vi "Measurement UI.vi"() -> ()   [LabVIEW 2024, in "Eff And Load Reg_Channel Ganging_UI.lvlib"]
uses:
  Eff And Load Reg_Channel Ganging_UI.lvlib
panel:
  in  "MeasGraphs":T1(tab)
  out "EfficiencyGraph":T2(graph)
  out "LoadRegulationGraph(V/A)":T3(graph)
  out "LoadRegulationGraph(%)":T3(graph)
  out "Load voltage deviation":dbl[](array[numeric])
  out "Ganged load voltages":dbl[](array[numeric])
  in  "Load current pole-zero ratio":dbl=0.3
  in  "Load current compensation frequency":dbl=180000.0
  in  "Load current gain bandwidth":dbl=14000.0
  in  "Source voltage pole-zero ratio":dbl=2.0
  in  "Source voltage compensation frequency":dbl=3530.0
  in  "Source voltage gain bandwidth":dbl=2000.0
  in  "Load slave resource names":string[](array[string])
  in  "Load master resource name":string
  in  "Source slave resource names":string[](array[string])
  in  "Source master resource name":string
  out "Load sweep points":i32
  out "Source sweep points":i32
  out "Voltage values":dbl[](array[numeric])
  out "Efficiency":dbl[](array[numeric])
  out "Ganged load currents":dbl[](array[numeric])
  in  "Mode of operation":T4(ring)=enum."Perform measurement" caption="MODE OF OPERATION"
  in  "MeasConfigurations":T5(tab)=enum."Source Config"
  in  "Nominal output voltage":dbl=1.0 caption="NOMINAL OUTPUT VOLTAGE" format="%.3fV"
  in  "Source delay":dbl=0.005 caption="SOURCE DELAY" format="%.3ps"
  in  "DUT setup time":dbl=1.0 caption="DUT SETUP TIME" format="%.3ps"
  in  "Aperture time":dbl=0.005 caption="APERTURE TIME" format="%.3ps"
  in  "PPSSlaveResourceNames":refnum<k15>[](array[refnum]) caption="SLAVE RESOURCE NAMES"
  in  "PPSMasterResourceName":refnum<k15> caption="MASTER RESOURCE NAME"
  in  "Source stop voltage":dbl=14.0 caption="VOLTAGE STOP LEVEL" format="%#_6pV"
  in  "Source transient response":i32(ring)=1038 caption="TRANSIENT RESPONSE" items=["Slow"=1041, "Normal"=1038, "Fast"=1039, "Custom"=1042]
  in  "Source sense":i32(ring)=1009 caption="SENSE" items=["Local"=1008, "Remote"=1009]
  in  "Source voltage level range":dbl=20.0 caption="VOLTAGE LEVEL RANGE" format="%#_6pV"
  in  "Source start voltage":dbl=6.0 caption="VOLTAGE START LEVEL" format="%#_6pV"
  in  "Source current limit high":dbl=25.0 caption="CURRENT LIMIT/LIMIT HIGH" format="%#_6pA"
  in  "Source current limit range":dbl=25.0 caption="CURRENT LIMIT RANGE" format="%#_6pA"
  in  "Source limit symmetry":enum32{"Symmetric", "Asymmetric"}(ring)=enum."Asymmetric" caption="LIMIT SYMMETRY"
  in  "Source current limit low":dbl=-0.6 caption="CURRENT LIMIT LOW" format="%#_6pA"
  in  "Source system configuration":enum32{"Series", "Parallel"}(ring)=enum."Parallel" caption="SYSTEM CONFIG"
  in  "Source compliance":string="Compliance"
  in  "Source sourceadapt":string="SourceAdapt"
  in  "Source voltage sweep points":i32=4 caption="NO. OF POINTS"
  in  "Source Custom Transient Response":bool
  out "Status":string
  in  "Load current sweep points/points per decade":i32=10 caption="PTS/PTS PER DECADE"
  in  "Load sweep type":string(combo)="Logarithmic" caption="SWEEP TYPE"
  in  "Load stop current":dbl=50.0 caption="CURRENT STOP LEVEL" format="%#_6pA"
  in  "Load sourceadapt":string="SourceAdapt"
  in  "Load compliance":string="Compliance"
  in  "Load system configuration":enum32{"Series", "Parallel"}(ring)=enum."Parallel" caption="SYSTEM CONFIG"
  in  "Load voltage limit low":dbl caption="VOLTAGE  LIMIT LOW" format="%#_6pV"
  in  "Load limit symmetry":enum32{"Symmetric", "Asymmetric"}(ring) caption="LIMIT SYMMETRY"
  in  "Load voltage limit range":dbl=6.0 caption="VOLTAGE LIMIT RANGE" format="%#_6pV"
  in  "Load voltage limit high":dbl=inf caption="VOLTAGE LIMIT/LIMIT HIGH" format="%#_6p"
  in  "Load start current":dbl=2.0 caption="CURRENT START LEVEL" format="%#_6pA"
  in  "Load current level range":dbl=80.0 caption="CURRENT LEVEL RANGE" format="%#_6pA"
  in  "Load sense":i32(ring)=1009 caption="SENSE" items=["Local"=1008, "Remote"=1009]
  in  "Load transient response":i32(ring)=1038 caption="TRANSIENT RESPONSE" items=["Slow"=1041, "Normal"=1038, "Fast"=1039, "Custom"=1042]
  in  "LoadSlaveResourceNames":refnum<k15>[](array[refnum]) caption="SLAVE RESOURCE NAMES"
  in  "LoadMasterResourceName":refnum<k15> caption="MASTER RESOURCE NAME"
  in  "Load Custom Transient Response":bool
  out "Status (Load)":string
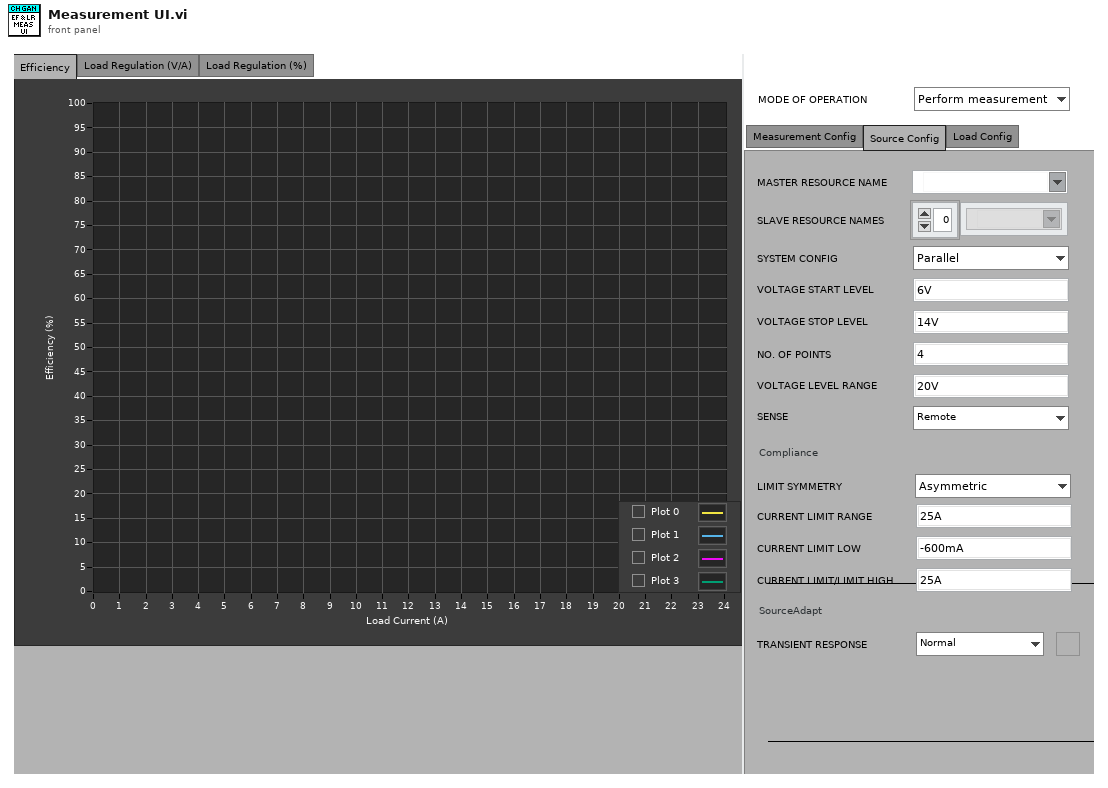
[diagram p1: front panel]
types:
  T1 = enum32{"Efficiency", "Load Regulation (V/A)", "Load Regulation (%)", "Hidden Controls"}
  T2 = cluster{"Ganged load currents":dbl[], "Efficiency":dbl[]}[]
  T3 = cluster{"Load currents":dbl[], "Efficiency":dbl[]}[]
  T4 = enum32{"Power on the DUT", "Perform measurement", "Power off the DUT"}
  T5 = enum32{"Measurement Config", "Source Config", "Load Config"}
  T6 = typedef "SourceAdapt Parameters.ctl" = cluster{"Voltage gain bandwidth":dbl, "Voltage compensation frequency":dbl, "Voltage pole-zero ratio":dbl, "Current gain bandwidth":dbl, "Current compensation frequency":dbl, "Current pole-zero ratio":dbl}
  T7 = cluster{"Ganged load currents":dbl[], "Efficiency":dbl[]}
  T8 = cluster{"Ganged load currents":dbl[], "Ganged load voltages":dbl[]}
  T9 = cluster{"Ganged load currents":dbl[], "Load voltage deviation":dbl[]}
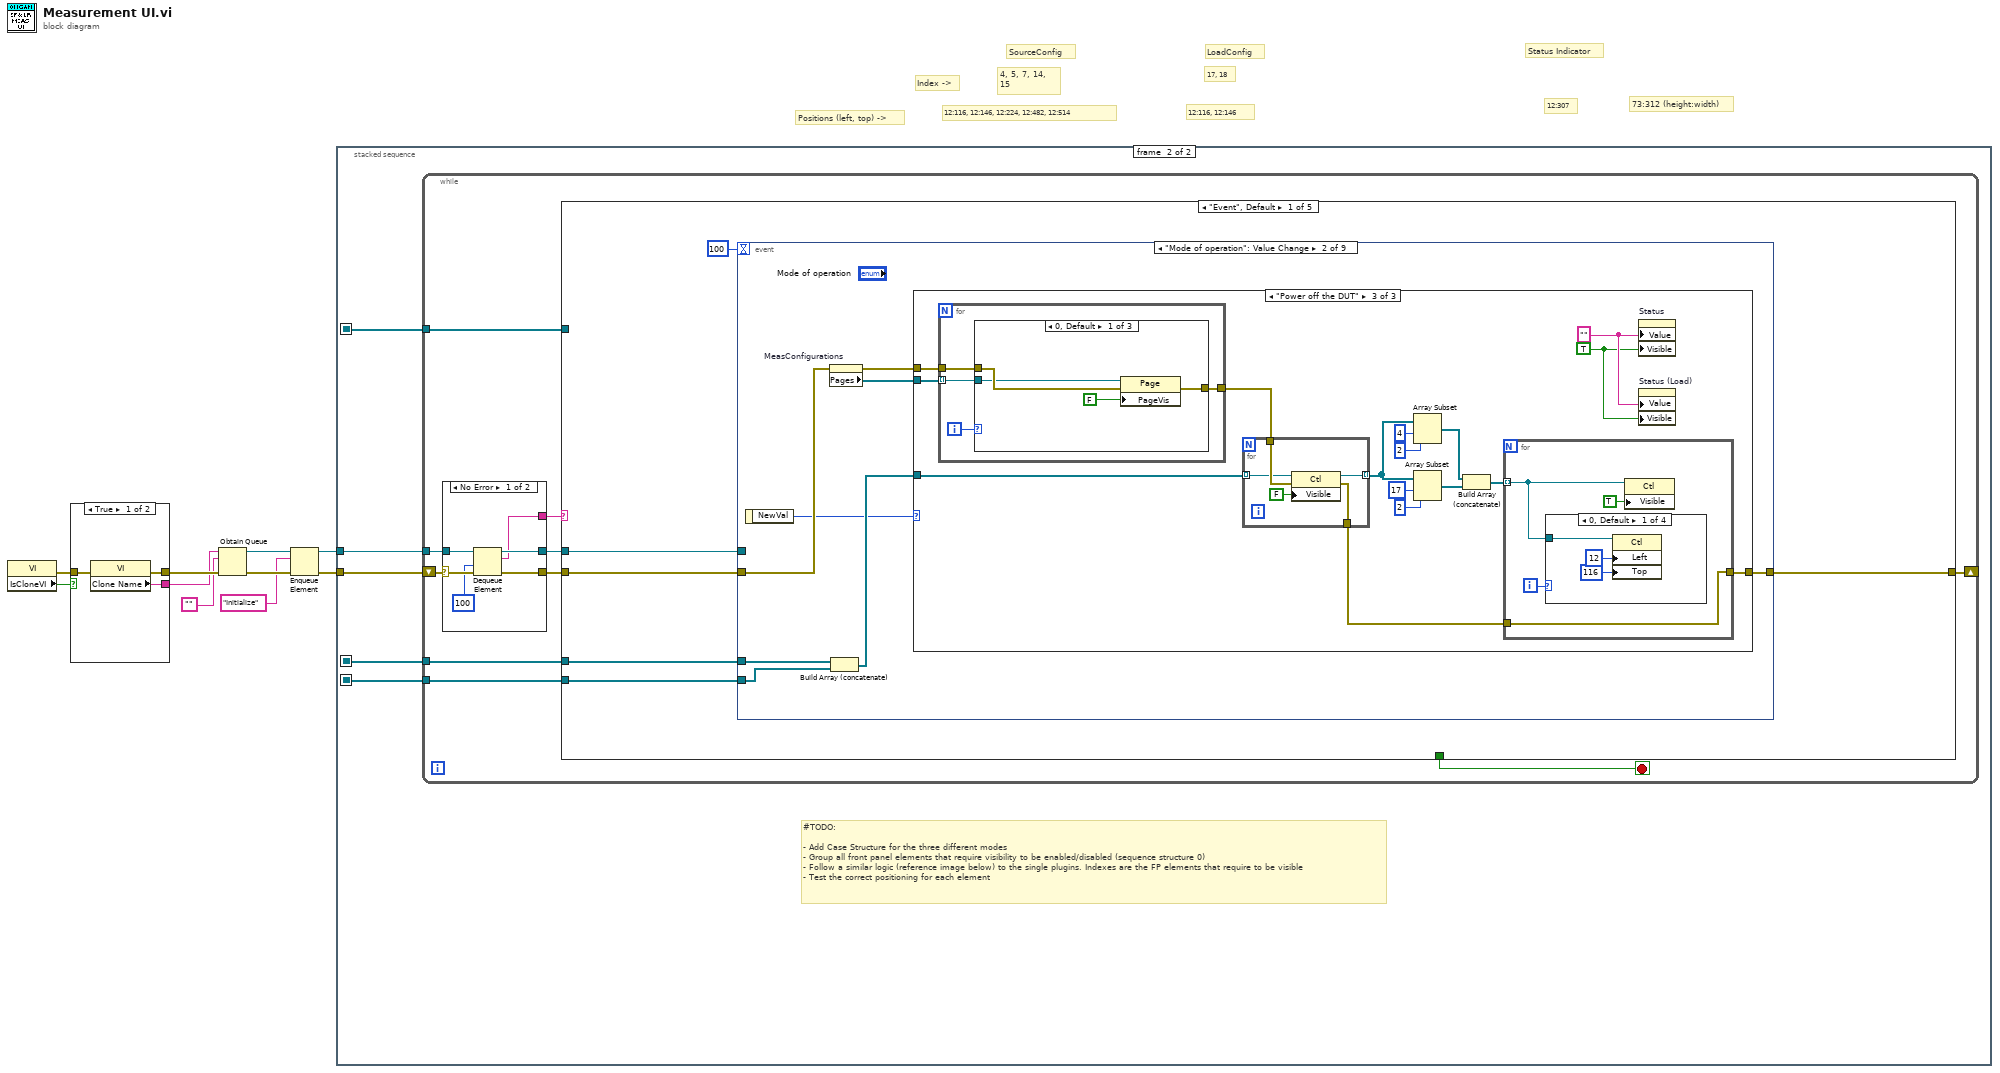
[diagram p0: block diagram]
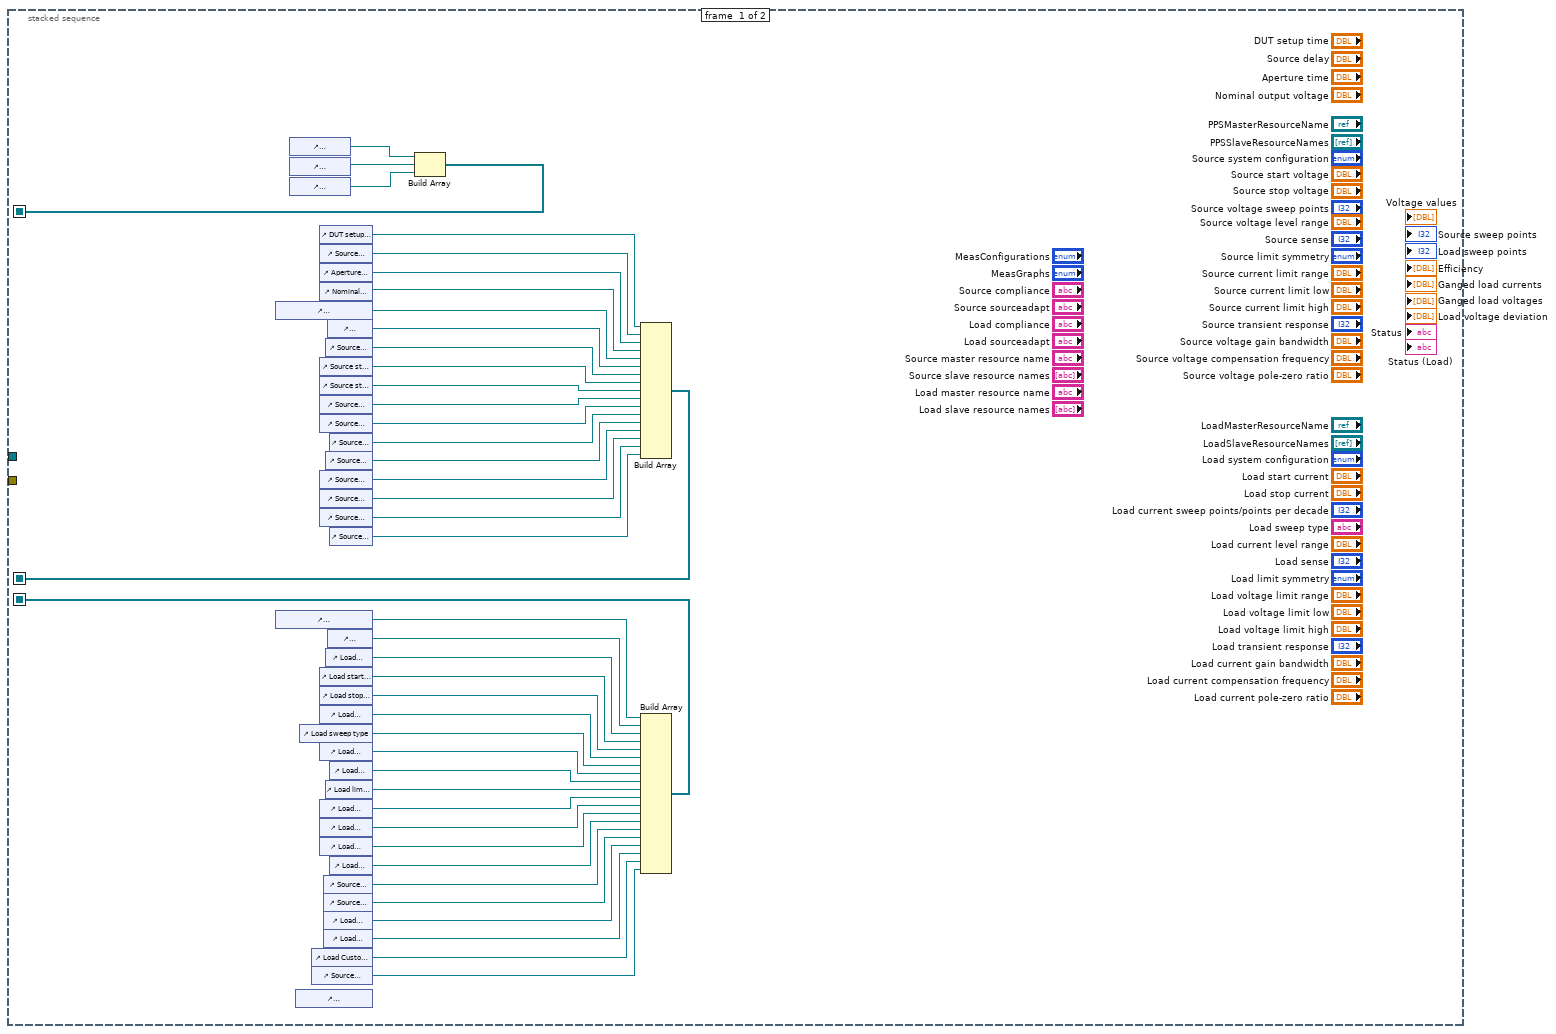
[diagram p2: hidden frame]
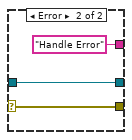
[diagram p3: hidden frame]
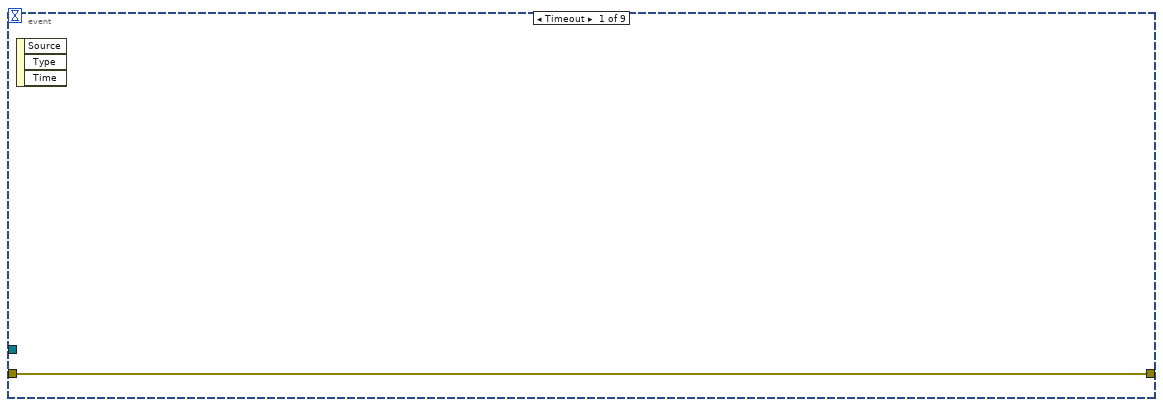
[diagram p4: hidden frame]
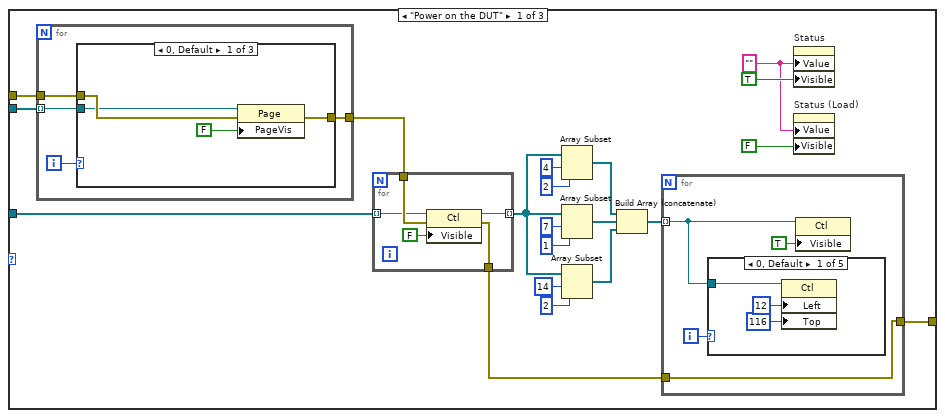
[diagram p5: hidden frame]
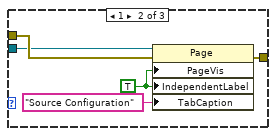
[diagram p6: hidden frame]
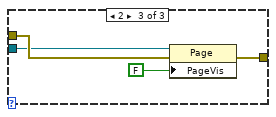
[diagram p7: hidden frame]
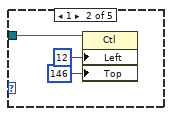
[diagram p8: hidden frame]
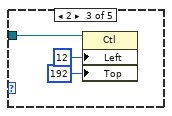
[diagram p9: hidden frame]
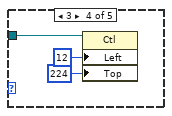
[diagram p10: hidden frame]
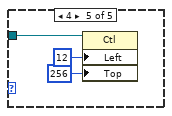
[diagram p11: hidden frame]
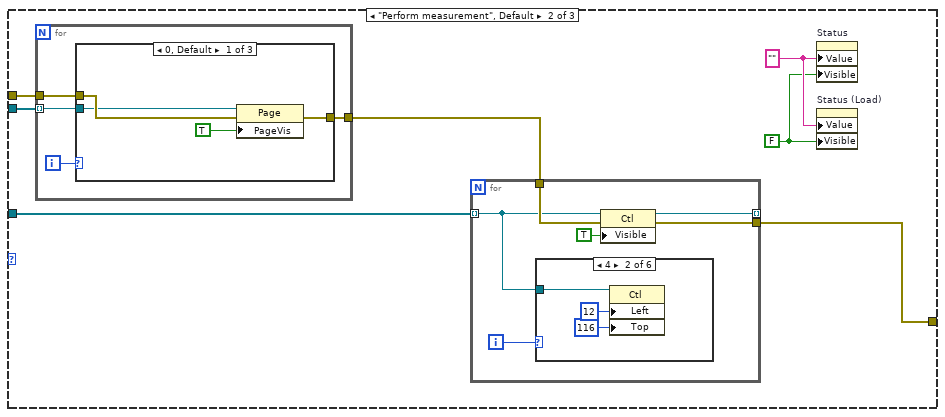
[diagram p12: hidden frame]
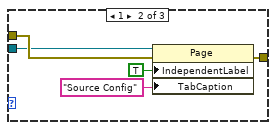
[diagram p13: hidden frame]
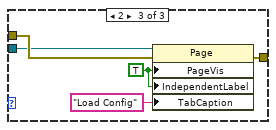
[diagram p14: hidden frame]
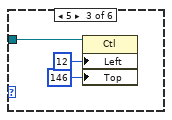
[diagram p16: hidden frame]
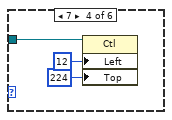
[diagram p17: hidden frame]
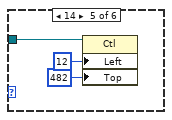
[diagram p18: hidden frame]
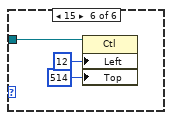
[diagram p19: hidden frame]
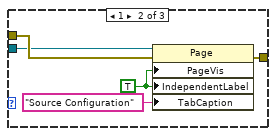
[diagram p20: hidden frame]
diagram:
  # "73:312 (height:width)"
  # "Status Indicator"
  # "Positions (left, top) ->"
  # "Index ->"
  # "LoadConfig"
  # "SourceConfig"
  # "12:307"
  # "12:116, 12:146"
  # "17, 18"
  # "12:116, 12:146, 12:224, 12:482, 12:514"
  # "4, 5, 7, 14, 15"
  n1 = property class="VI"() -> (error out=w1:errorcluster, "IsCloneVI"=w2:bool)  [unwired: 2 in, 1 out]
  n2 = case shown="True" w2 {
    tunnel: [w13 w16] -> w10
    tunnel: [w12 w15] -> w9
    tunnel: w1 -> [w11 w14]
    frame True {
      n3 = property class="VI"(error in=w11) -> (error out=w13:errorcluster, "Clone Name"=w12:string)  [unwired: 1 in, 1 out]
    }
    frame False {
      n4 = property class="VI"(error in=w14) -> (error out=w16:errorcluster, "Name"=w15:string)  [unwired: 1 in, 1 out]
    }
  }
  n5 = Obtain Queue(name (unnamed)=w9, element data type="", error in (no error)=w10) -> (queue out=w6:refnum<queue>, error out=w8:errorcluster)  [unwired: 2 in, 1 out]
  n6 = Enqueue Element(queue=w6, element="Initialize", error in (no error)=w8) -> (queue out=w5:refnum<queue>, error out=w7:errorcluster)  [unwired: 1 in, 1 out]
  n7 = stacked-sequence {
    seq-local: [w56 _] -> [_ w62]
    seq-local: [w24 _] -> [_ w61]
    seq-local: [w23 _] -> [_ w60]
    tunnel: w7 -> [_ w64]
    tunnel: w5 -> [_ w63]
    frame #0 {
      n8 = control-ref of="PPSMasterResourceName"() -> (w51:refnum<vi>)
      n9 = control-ref of="LoadMasterResourceName"() -> (w38:refnum<vi>)
      n10 = control-ref of="EfficiencyGraph"() -> (w59:refnum<vi>)
      n11 = control-ref of="LoadRegulationGraph(V/A)"() -> (w58:refnum<vi>)
      n12 = control-ref of="LoadRegulationGraph(%)"() -> (w57:refnum<vi>)
      n13 = control-ref of="MeasConfigurations"() -> ()  [unwired: 1 out]
      n14 = control-ref of="Load sweep type"() -> (w25:refnum<vi>)
      n15 = control-ref of="Load Custom Transient Response"() -> (w18:refnum<vi>)
      n16 = control-ref of="Source Custom Transient Response"() -> (w17:refnum<vi>)
      n17 = control-ref of="DUT setup time"() -> (w55:refnum<vi>)
      n18 = control-ref of="Source delay"() -> (w54:refnum<vi>)
      n19 = control-ref of="Aperture time"() -> (w53:refnum<vi>)
      n20 = control-ref of="Nominal output voltage"() -> (w52:refnum<vi>)
      n21 = control-ref of="Source start voltage"() -> (w48:refnum<vi>)
      n22 = control-ref of="Source stop voltage"() -> (w47:refnum<vi>)
      n23 = control-ref of="Source voltage sweep points"() -> (w39:refnum<vi>)
      n24 = control-ref of="Source voltage level range"() -> (w40:refnum<vi>)
      n25 = control-ref of="Source current limit range"() -> (w43:refnum<vi>)
      n26 = control-ref of="Source current limit low"() -> (w44:refnum<vi>)
      n27 = control-ref of="Source current limit high"() -> (w45:refnum<vi>)
      n28 = control-ref of="Load start current"() -> (w35:refnum<vi>)
      n29 = control-ref of="Load stop current"() -> (w29:refnum<vi>)
      n30 = control-ref of="Load current sweep points/points per decade"() -> (w27:refnum<vi>)
      n31 = control-ref of="Load current level range"() -> (w26:refnum<vi>)
      n32 = control-ref of="Load voltage limit range"() -> (w31:refnum<vi>)
      n33 = control-ref of="Load voltage limit low"() -> (w32:refnum<vi>)
      n34 = control-ref of="Load voltage limit high"() -> (w33:refnum<vi>)
      n35 = control-ref of="Source compliance"() -> (w19:refnum<vi>)
      n36 = control-ref of="Source sourceadapt"() -> (w20:refnum<vi>)
      n37 = control-ref of="Load compliance"() -> (w21:refnum<vi>)
      n38 = control-ref of="Load sourceadapt"() -> (w22:refnum<vi>)
      n39 = control-ref of="Source system configuration"() -> (w49:refnum<vi>)
      n40 = control-ref of="Source limit symmetry"() -> (w42:refnum<vi>)
      n41 = control-ref of="Load system configuration"() -> (w36:refnum<vi>)
      n42 = control-ref of="Load limit symmetry"() -> (w30:refnum<vi>)
      n43 = control-ref of="PPSSlaveResourceNames"() -> (w50:refnum<vi>)
      n44 = control-ref of="LoadSlaveResourceNames"() -> (w37:refnum<vi>)
      n45 = control-ref of="Source sense"() -> (w41:refnum<vi>)
      n46 = control-ref of="Source transient response"() -> (w46:refnum<vi>)
      n47 = control-ref of="Load sense"() -> (w28:refnum<vi>)
      n48 = control-ref of="Load transient response"() -> (w34:refnum<vi>)
      n49 = Build Array(w59, w58, w57) -> (w56:refnum<vi>[])
      n50 = Build Array(w55, w54, w53, w52, w51, w50, w49, w48, w47, w39, w40, w41, w42, w43, w44, w45, w46) -> (w24:refnum<vi>[])
      n51 = Build Array(w38, w37, w36, w35, w29, w27, w25, w26, w28, w30, w31, w32, w33, w34, w19, w20, w21, w22, w18, w17) -> (w23:refnum<vi>[])
    }
    frame #1 {
      # "#TODO:\n\n- Add Case Structure for the three different modes\n- Group all front panel elements that require visibility to be enabled/disabled (sequence structure 0)\n- Follow a similar logic (reference image below) to the single plugins. Indexes are the FP elements that require to be visible\n- Test the correct positioning for each element"
      n52 = while {
        shift-right: [w69] -> _
        shift-left: w64 -> [w74]
        tunnel: w63 -> [w72]
        tunnel: w62 -> [w67]
        tunnel: w61 -> [w66]
        tunnel: w60 -> [w65]
        stop <- w68 stop-if-true
        n53 = case shown="No Error" w74 {
          selector: w74 -> [w80 w83]
          tunnel: [w79 w83] -> w73
          tunnel: w72 -> [w78 w82]
          tunnel: [w77 w82] -> w71
          tunnel: [w76 "Handle Error"] -> w70
          frame No Error {
            n54 = Dequeue Element(queue=w78, timeout in ms (-1)=100, error in (no error)=w80) -> (queue out=w77:refnum<queue>, element=w76:string, error out=w79:errorcluster)  [unwired: 1 out]
          }
          frame Error {
          }
        }
        n55 = case shown="\"Event\", Default" w70 {
          tunnel: w73 -> [w88 w284 w299 w356 w357]
          tunnel: w71 -> [w86 _ _ w354 _]
          tunnel: [w89 w284 w299 w351 w357] -> w69
          tunnel: [_ _ _ TRUE _] -> w68
          tunnel: w67 -> [_ _ w287 _ _]
          tunnel: w66 -> [w85 _ _ _ _]
          tunnel: w65 -> [w84 _ _ _ _]
          frame "Event", Default {
            n56 = event shown="[1] \"Mode of operation\": Value Change" {
              selector: _ -> [_ _ _ _ _ _ _ _ _]
              dyn-events: _ -> [_ _ _ _ _ _ _ _ _]
              timeout: 100 -> [_ _ _ _ _ _ _ _ _]
              tunnel: [w90 w91 w262 w264 w265 w267 w272 w277 w281] -> w89
              tunnel: w88 -> [w90 w98 w262 w264 w265 w267 w272 w277 w282]
              tunnel: w86 -> [_ _ _ _ _ _ _ _ w280]
              tunnel: w85 -> [_ w95 _ _ _ _ _ _ _]
              tunnel: w84 -> [_ w94 _ _ _ _ _ _ _]
              event Timeout {
                n57 = event-data() -> ()  [unwired: 1 in, 3 out]
              }
              event "Mode of operation": Value Change {
                n58 = event-data() -> ("NewVal"=w96:T4)  [unwired: 1 in]
                n59 = property on="MeasConfigurations" class="TabCtl (strict)"(error in=w98) -> (error out=w92:errorcluster, "Pages"=w93:refnum<vi>[])  [unwired: 1 in, 1 out]
                n60 = Build Array (concatenate)(w95, w94) -> (w97:refnum<vi>[])
                n61 = case shown="\"Power off the DUT\"" w96 {
                  tunnel: w97 -> [w118 w166 w221]
                  tunnel: w93 -> [w106 w165 w216]
                  tunnel: w92 -> [w105 w164 w215]
                  tunnel: [w102 w162 w212] -> w91
                  frame "Power on the DUT" {
                    w100 = ""
                    n62 = for {
                      tunnel: w106 -> [w121] mode=indexing
                      tunnel: w105 -> [w120]
                      tunnel: [w119] -> w104
                      i -> [w122]
                      n63 = case shown="0, Default" w122 {
                        tunnel: w121 -> [w125 w130 w134]
                        tunnel: w120 -> [w126 w131 w135]
                        tunnel: [w123 w128 w132] -> w119
                        frame 0, Default {
                          n64 = property class="Page"(reference=w125, error in=w126, "PageVis"=FALSE ("Independent Label")) -> (error out=w123:errorcluster)  [unwired: 1 out]
                        }
                        frame 1 {
                          w127 = TRUE ("Independent Label")
                          n65 = property class="Page"(reference=w130, error in=w131, "PageVis"=w127, "IndependentLabel"=w127, "TabCaption"="Source Configuration" ("Tab Caption")) -> (error out=w128:errorcluster)  [unwired: 1 out]
                        }
                        frame 2 {
                          n66 = property class="Page"(reference=w134, error in=w135, "PageVis"=FALSE ("Independent Label")) -> (error out=w132:errorcluster)  [unwired: 1 out]
                        }
                      }
                    }
                    n67 = for {
                      tunnel: w118 -> [w158] mode=indexing
                      tunnel: [w156] -> w111 mode=indexing
                      tunnel: w104 -> [w159]
                      tunnel: [w155] -> w103
                      n68 = property class="Ctl"(reference=w158, error in=w159, "Visible"=FALSE) -> (reference out=w156:refnum<vi>, error out=w155:errorcluster)
                    }
                    n69 = Array Subset(array=w111, index=4, length=2) -> (w109:refnum<vi>[])
                    n70 = Array Subset(array=w111, index=7, length=1) -> (w110:refnum<vi>[])
                    n71 = Array Subset(array=w111, index=14, length=2) -> (w108:refnum<vi>[])
                    n72 = Build Array (concatenate)(w109, w110, w108) -> (w107:refnum<vi>[])
                    n73 = for {
                      tunnel: w107 -> [w137] mode=indexing
                      tunnel: w103 -> [w136]
                      tunnel: [w136] -> w102
                      i -> [w138]
                      n74 = case shown="0, Default" w138 {
                        tunnel: w137 -> [w142 w145 w148 w151 w154]
                        frame 0, Default {
                          n75 = property class="Ctl"(reference=w142, "Left"=12 ("Position:Left"), "Top"=116 ("Position:Left")) -> ()  [unwired: 1 in, 2 out]
                        }
                        frame 1 {
                          n76 = property class="Ctl"(reference=w145, "Left"=12 ("Position:Left"), "Top"=146 ("Position:Left")) -> ()  [unwired: 1 in, 2 out]
                        }
                        frame 2 {
                          n77 = property class="Ctl"(reference=w148, "Left"=12 ("Position:Left"), "Top"=192 ("Position:Left")) -> ()  [unwired: 1 in, 2 out]
                        }
                        frame 3 {
                          n78 = property class="Ctl"(reference=w151, "Left"=12 ("Position:Left"), "Top"=224 ("Position:Left")) -> ()  [unwired: 1 in, 2 out]
                        }
                        frame 4 {
                          n79 = property class="Ctl"(reference=w154, "Left"=12 ("Position:Left"), "Top"=256 ("Position:Left")) -> ()  [unwired: 1 in, 2 out]
                        }
                      }
                      n80 = property class="Ctl"(reference=w137, "Visible"=TRUE) -> ()  [unwired: 1 in, 2 out]
                    }
                    n81 = property on="Status" class="Str"("Value"=w100, "Visible"=TRUE) -> ()  [unwired: 2 in, 2 out]
                    n82 = property on="Status (Load)" class="Str"("Value"=w100, "Visible"=FALSE) -> ()  [unwired: 2 in, 2 out]
                  }
                  frame "Perform measurement", Default {
                    w160 = FALSE ("Visible")
                    w161 = ""
                    n83 = for {
                      tunnel: w165 -> [w169] mode=indexing
                      tunnel: w164 -> [w168]
                      tunnel: [w167] -> w163
                      i -> [w170]
                      n84 = case shown="0, Default" w170 {
                        tunnel: w169 -> [w173 w178 w183]
                        tunnel: w168 -> [w174 w179 w184]
                        tunnel: [w171 w175 w182] -> w167
                        frame 0, Default {
                          n85 = property class="Page"(reference=w173, error in=w174, "PageVis"=TRUE ("Independent Label")) -> (error out=w171:errorcluster)  [unwired: 1 out]
                        }
                        frame 1 {
                          n86 = property class="Page"(reference=w178, error in=w179, "IndependentLabel"=TRUE ("Independent Label"), "TabCaption"="Source Config" ("Tab Caption")) -> (error out=w175:errorcluster)  [unwired: 1 out]
                        }
                        frame 2 {
                          w181 = TRUE ("Independent Label")
                          n87 = property class="Page"(reference=w183, error in=w184, "PageVis"=w181, "IndependentLabel"=w181, "TabCaption"="Load Config" ("Tab Caption")) -> (error out=w182:errorcluster)  [unwired: 1 out]
                        }
                      }
                    }
                    n88 = for {
                      tunnel: w166 -> [w186] mode=indexing
                      tunnel: [w188] -> _ mode=indexing
                      tunnel: w163 -> [w190]
                      tunnel: [w185] -> w162
                      i -> [w187]
                      n89 = case shown="4" w187 {
                        tunnel: w186 -> [_ w193 w196 w199 w202 w205]
                        frame 0, Default {
                        }
                        frame 4 {
                          n90 = property class="Ctl"(reference=w193, "Left"=12 ("Position:Left"), "Top"=116 ("Position:Left")) -> ()  [unwired: 1 in, 2 out]
                        }
                        frame 5 {
                          n91 = property class="Ctl"(reference=w196, "Left"=12 ("Position:Left"), "Top"=146 ("Position:Left")) -> ()  [unwired: 1 in, 2 out]
                        }
                        frame 7 {
                          n92 = property class="Ctl"(reference=w199, "Left"=12 ("Position:Left"), "Top"=224 ("Position:Left")) -> ()  [unwired: 1 in, 2 out]
                        }
                        frame 14 {
                          n93 = property class="Ctl"(reference=w202, "Left"=12 ("Position:Left"), "Top"=482 ("Position:Left")) -> ()  [unwired: 1 in, 2 out]
                        }
                        frame 15 {
                          n94 = property class="Ctl"(reference=w205, "Left"=12 ("Position:Left"), "Top"=514 ("Position:Left")) -> ()  [unwired: 1 in, 2 out]
                        }
                      }
                      n95 = property class="Ctl"(reference=w186, error in=w190, "Visible"=TRUE) -> (reference out=w188:refnum<vi>, error out=w185:errorcluster)
                    }
                    n96 = property on="Status" class="Str"("Value"=w161, "Visible"=w160) -> ()  [unwired: 2 in, 2 out]
                    n97 = property on="Status (Load)" class="Str"("Value"=w161, "Visible"=w160) -> ()  [unwired: 2 in, 2 out]
                  }
                  frame "Power off the DUT" {
                    w206 = TRUE
                    w207 = ""
                    n98 = for {
                      tunnel: w216 -> [w224] mode=indexing
                      tunnel: w215 -> [w223]
                      tunnel: [w222] -> w214
                      i -> [w225]
                      n99 = case shown="0, Default" w225 {
                        tunnel: w224 -> [w228 w233 w238]
                        tunnel: w223 -> [w229 w234 w239]
                        tunnel: [w226 w231 w236] -> w222
                        frame 0, Default {
                          n100 = property class="Page"(reference=w228, error in=w229, "PageVis"=FALSE ("Independent Label")) -> (error out=w226:errorcluster)  [unwired: 1 out]
                        }
                        frame 1 {
                          w230 = TRUE ("Independent Label")
                          n101 = property class="Page"(reference=w233, error in=w234, "PageVis"=w230, "IndependentLabel"=w230, "TabCaption"="Source Configuration" ("Tab Caption")) -> (error out=w231:errorcluster)  [unwired: 1 out]
                        }
                        frame 2 {
                          w235 = TRUE ("Independent Label")
                          n102 = property class="Page"(reference=w238, error in=w239, "PageVis"=w235, "IndependentLabel"=w235, "TabCaption"="Load Configuration" ("Tab Caption")) -> (error out=w236:errorcluster)  [unwired: 1 out]
                        }
                      }
                    }
                    n103 = for {
                      tunnel: w221 -> [w259] mode=indexing
                      tunnel: [w257] -> w209 mode=indexing
                      tunnel: w214 -> [w260]
                      tunnel: [w256] -> w213
                      n104 = property class="Ctl"(reference=w259, error in=w260, "Visible"=FALSE) -> (reference out=w257:refnum<vi>, error out=w256:errorcluster)
                    }
                    n105 = Array Subset(array=w209, index=4, length=2) -> (w218:refnum<vi>[])
                    n106 = Array Subset(array=w209, index=17, length=2) -> (w208:refnum<vi>[])
                    n107 = Build Array (concatenate)(w218, w208) -> (w217:refnum<vi>[])
                    n108 = for {
                      tunnel: w217 -> [w241] mode=indexing
                      tunnel: w213 -> [w240]
                      tunnel: [w240] -> w212
                      i -> [w242]
                      n109 = case shown="0, Default" w242 {
                        tunnel: w241 -> [w246 w249 w252 w255]
                        frame 0, Default {
                          n110 = property class="Ctl"(reference=w246, "Left"=12 ("Position:Left"), "Top"=116 ("Position:Left")) -> ()  [unwired: 1 in, 2 out]
                        }
                        frame 1 {
                          n111 = property class="Ctl"(reference=w249, "Left"=12 ("Position:Left"), "Top"=146 ("Position:Left")) -> ()  [unwired: 1 in, 2 out]
                        }
                        frame 2 {
                          n112 = property class="Ctl"(reference=w252, "Left"=12 ("Position:Left"), "Top"=116 ("Position:Left")) -> ()  [unwired: 1 in, 2 out]
                        }
                        frame 3 {
                          n113 = property class="Ctl"(reference=w255, "Left"=12 ("Position:Left"), "Top"=146 ("Position:Left")) -> ()  [unwired: 1 in, 2 out]
                        }
                      }
                      n114 = property class="Ctl"(reference=w241, "Visible"=TRUE) -> ()  [unwired: 1 in, 2 out]
                    }
                    n115 = property on="Status" class="Str"("Value"=w207, "Visible"=w206) -> ()  [unwired: 2 in, 2 out]
                    n116 = property on="Status (Load)" class="Str"("Value"=w207, "Visible"=w206) -> ()  [unwired: 2 in, 2 out]
                  }
                }
              }
              event "PPSMasterResourceName": Value Change {
                n117 = event-data() -> ("NewVal"=w261:refnum<k15>)  [unwired: 1 in]
                n118 = property on="Source master resource name" class="Str"("Value"=w261) -> ()  [unwired: 2 in, 2 out]
              }
              event "PPSSlaveResourceNames": Value Change {
                n119 = event-data() -> ("NewVal"=w263:refnum<k15>[])  [unwired: 1 in]
                n120 = property on="Source slave resource names" class="Arr (strict)"("Value"=w263) -> ()  [unwired: 2 in, 2 out]
              }
              event "LoadMasterResourceName": Value Change {
                n121 = event-data() -> ("NewVal"=w266:refnum<k15>)  [unwired: 1 in]
                n122 = property on="Load master resource name" class="Str"("Value"=w266) -> ()  [unwired: 2 in, 2 out]
              }
              event "LoadSlaveResourceNames": Value Change {
                n123 = event-data() -> ("NewVal"=w268:refnum<k15>[])  [unwired: 1 in]
                n124 = property on="Load slave resource names" class="Arr (strict)"("Value"=w268) -> ()  [unwired: 2 in, 2 out]
              }
              event "Source Custom Transient Response": Value Change {
                n125 = event-data() -> ()  [unwired: 1 in, 6 out]
                n126 = call "Custom Transient Response for Sweep & Single Point.vi"() -> ("SourceAdapt Parameters"=w273:T6)  [unwired: 11 in]
                n127 = Unbundle By Name(w273) -> ("Voltage gain bandwidth"=w270:dbl, "Voltage compensation frequency"=w271:dbl, "Voltage pole-zero ratio"=w269:dbl)
                n128 = property on="Source voltage gain bandwidth" class="DigNum (strict)"("Value"=w270) -> ()  [unwired: 2 in, 2 out]
                n129 = property on="Source voltage compensation frequency" class="DigNum (strict)"("Value"=w271) -> ()  [unwired: 2 in, 2 out]
                n130 = property on="Source voltage pole-zero ratio" class="DigNum (strict)"("Value"=w269) -> ()  [unwired: 2 in, 2 out]
              }
              event "Load Custom Transient Response": Value Change {
                n131 = event-data() -> ()  [unwired: 1 in, 6 out]
                n132 = call "Custom Transient Response for Sweep & Single Point.vi"() -> ("SourceAdapt Parameters"=w278:T6)  [unwired: 11 in]
                n133 = Unbundle By Name(w278) -> ("Current gain bandwidth"=w274:dbl, "Current compensation frequency"=w276:dbl, "Current pole-zero ratio"=w275:dbl)
                n134 = property on="Load current gain bandwidth" class="DigNum (strict)"("Value"=w274) -> ()  [unwired: 2 in, 2 out]
                n135 = property on="Load current compensation frequency" class="DigNum (strict)"("Value"=w276) -> ()  [unwired: 2 in, 2 out]
                n136 = property on="Load current pole-zero ratio" class="DigNum (strict)"("Value"=w275) -> ()  [unwired: 2 in, 2 out]
              }
              event Panel Close? {
                n137 = event-data() -> ()  [unwired: 1 in, 4 out]
                n138 = Enqueue Element(queue=w280, element="Exit", error in (no error)=w282) -> (error out=w281:errorcluster)  [unwired: 1 in, 2 out]
                n139 = event-data("Discard?"=TRUE) -> ()  [unwired: 1 in, 1 out]
              }
            }
          }
          frame "Initialize" {
          }
          frame "Post UI Update" {
            w294 = u32[] [15787074, 5682409, 15535092, 40563, 13983232, 35009, 15113984, 13400487, 15993633, 10221451, 8148942, 15869817, 32914, 10196480, 6271923, 16355671]  # Plot colors
            # "This case will be triggered, after framework updates the User interface with result values."
            n140 = local read "Source sweep points"() -> (w292:i32)
            n141 = local read "Voltage values"() -> (w293:dbl[])
            n142 = for {
              tunnel: w294 -> [w304]
              tunnel: w287 -> [w303] mode=indexing
              tunnel: w293 -> [w302]
              tunnel: w292 -> [w301]
              tunnel: [w300] -> w286
              n143 = for {
                tunnel: w302 -> [w317] mode=indexing
                tunnel: [w317] -> w300 mode=indexing
                tunnel: w303 -> [w310]
                tunnel: w301 -> [w307]
                tunnel: w304 -> [w313] mode=indexing
                i -> [w311]
                n144 = Greater?(x=w311, y=3) -> (0:w315:bool)
                n145 = To Unsigned Long Integer(number=w311) -> (unsigned 32bit integer=w314:u32)
                n146 = Increment(x=w311) -> (x+1=w309:i32)
                n147 = Format Value(format string="%.3f", value (0)=w317) -> (output string=w320:string)  [unwired: 1 out]
                n148 = case shown="False" w315 {
                  tunnel: w310 -> [w326 w332]
                  tunnel: w309 -> [w325 _]
                  tunnel: [w324 w331] -> w308
                  tunnel: w307 -> [w322 w327]
                  tunnel: [w323 w330] -> w306
                  frame False {
                    n149 = property on="Property Node" class="XYGraph (strict)"(reference=w326, "LegScrollVis"=FALSE ("Legend:Scrollbar Visible"), "LegNumRows"=w325, "LegPlotMin"=w322) -> (reference out=w324:refnum<vi>, error out=w323:errorcluster)  [unwired: 1 in]
                  }
                  frame True {
                    n150 = property on="Property Node" class="XYGraph (strict)"(reference=w332, "LegScrollVis"=TRUE ("Legend:Scrollbar Visible"), "LegNumRows"=u32 4 ("Legend:Number of Rows"), "LegPlotMin"=w327) -> (reference out=w331:refnum<vi>, error out=w330:errorcluster)  [unwired: 1 in]
                  }
                }
                n151 = Concatenate Strings(" Vin = " ("string"), w320) -> (w305:string)
                n152 = property on="Property Node" class="XYGraph (strict)"(reference=w308, error in=w306, "Active Plot"=w314, "Plot.Point Style"=u8 5, "Plot.Plot Color"=w313, "Plot.Fill/Pt. Color"=w313, "Plot.Plot Name"=w305) -> ()  [unwired: 2 out]
              }
            }
            n153 = local read "Load voltage deviation"() -> (w290:dbl[])
            n154 = local read "Ganged load currents"() -> (w298:dbl[])
            n155 = local read "Ganged load voltages"() -> (w291:dbl[])
            n156 = local read "Load sweep points"() -> (w295:i32)
            n157 = Array Size(array=w286) -> (size(s)=w285:i32)
            n158 = local read "Efficiency"() -> (w297:dbl[])
            n159 = for {
              N: w285 -> [_]
              tunnel: [w349] -> w296 mode=indexing
              shift-right: [w348] -> _
              shift-left: w298 -> [w346]
              shift-right: [w344] -> _
              shift-left: w297 -> [w345]
              tunnel: w295 -> [w343]
              shift-right: [w340] -> _
              shift-left: w291 -> [w342]
              shift-right: [w337] -> _
              shift-left: w290 -> [w341]
              tunnel: [w336] -> w288 mode=indexing
              tunnel: [w335] -> w289 mode=indexing
              w334 = 0 ("index")
              n160 = Delete From Array(array=w346, length=w343, index=w334) -> (deleted portion=w338:dbl[], array with subset deleted=w348:dbl[])
              n161 = Delete From Array(array=w345, length=w343, index=w334) -> (deleted portion=w347:dbl[], array with subset deleted=w344:dbl[])
              n162 = Delete From Array(array=w342, length=w343, index=w334) -> (deleted portion=w339:dbl[], array with subset deleted=w340:dbl[])
              n163 = Delete From Array(array=w341, length=w343, index=w334) -> (deleted portion=w333:dbl[], array with subset deleted=w337:dbl[])
              n164 = Bundle("Ganged load currents"=w338, "Efficiency"=w347) -> (w349:T7)  [unwired: 1 in]
              n165 = Bundle("Ganged load currents"=w338, "Ganged load voltages"=w339) -> (w335:T8)  [unwired: 1 in]
              n166 = Bundle("Ganged load currents"=w338, "Load voltage deviation"=w333) -> (w336:T9)  [unwired: 1 in]
            }
            "EfficiencyGraph" <- w296
            "LoadRegulationGraph(V/A)" <- w289
            "LoadRegulationGraph(%)" <- w288
          }
          frame "Exit" {
            # "This case is triggered to close the User Interface from framework"
            n167 = Flush Queue(queue=w354, error in (no error)=w356) -> (queue out=w353:refnum<queue>, error out=w352:errorcluster)  [unwired: 1 out]
            n168 = Release Queue(queue=w353, force destroy? (F)=TRUE, error in (no error)=w352) -> (error out=w351:errorcluster)  [unwired: 2 out]
          }
          frame "Handle Error" {
          }
        }
      }
    }
  }
